vi "DIGITIZER_ADD_TEGAM_SCALING.vi"(1 "TEGAM SCALING PRESENT?":bool, 2 "DIGITIZER 2 WAVEFORM":T1(array[cluster]), 3 "Channel1 Scale":dbl, 4 "DIGITIZER 1 WAVEFORM":T1(array[cluster])) -> (0 "WAVEFORMS OUT":T1(array[cluster]))   [LabVIEW 2010]
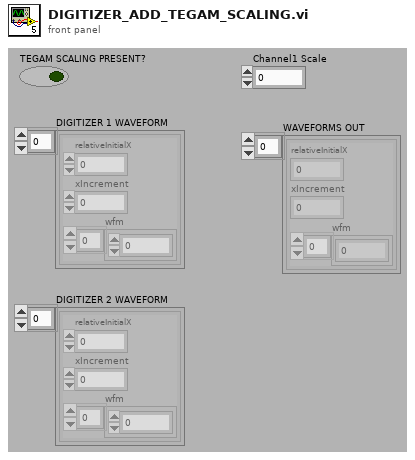
[diagram p1: front panel]
types:
  T1 = cluster{"relativeInitialX":dbl, "xIncrement":dbl, "wfm":dbl[]}[]
  T2 = cluster{"relativeInitialX":dbl, "xIncrement":dbl, "wfm":dbl[]}
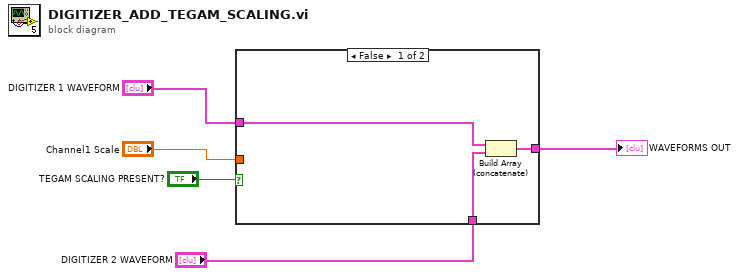
[diagram p0: block diagram]
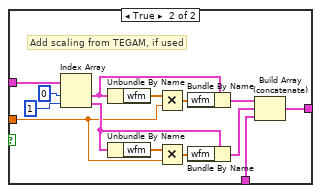
[diagram p2: hidden frame]
diagram:
  n1 = case shown="False" "TEGAM SCALING PRESENT?" {
    tunnel: "DIGITIZER 1 WAVEFORM" -> [w8 w22]
    tunnel: "Channel1 Scale" -> [_ w9]
    tunnel: "DIGITIZER 2 WAVEFORM" -> [w7 w15]
    tunnel: [w6 w14] -> w4
    frame False {
      n2 = Build Array (concatenate)(w8, w7) -> (w6:T1)
    }
    frame True {
      # "Add scaling from TEGAM, if used"
      n3 = Index Array(array=w22, index #1=0 ("index"), index #2=1 ("index")) -> (element #1=w19:T2, element #2=w11:T2)
      n4 = Unbundle By Name(w19) -> ("wfm"=w21:dbl[])
      n5 = Unbundle By Name(w11) -> ("wfm"=w13:dbl[])
      n6 = Multiply(x=w21, y=w9) -> (x*y=w18:dbl[])
      n7 = Multiply(x=w13, y=w9) -> (x*y=w12:dbl[])
      n8 = Bundle By Name(cluster=w19, "wfm"=w18) -> (w16:T2)
      n9 = Bundle By Name(cluster=w11, "wfm"=w12) -> (w10:T2)
      n10 = Build Array (concatenate)(w16, w10, w15) -> (w14:T1)
    }
  }
  "WAVEFORMS OUT" <- w4
